vi "Get Wire Type.vi"(8 "error in (no error)":errorcluster, 11 "Message in":refnum<class "Raw Message.lvclass">) -> (0 "error out":errorcluster, 2 "Wire Type":T1, 3 "Message out":refnum<class "Raw Message.lvclass">)   [LabVIEW 2020, in "Protobuf RAW.lvlib" / "Raw Message.lvclass"]
uses:
  Raw Message.lvclass
  Type Serializer/Wire Type.ctl
  Raw Message.lvclass/Raw Message.ctl
  Wire Type Group/Wire Type Group.lvclass
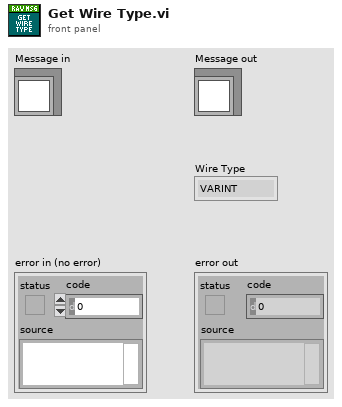
[diagram p1: front panel]
types:
  T1 = typedef "Protobuf RAW.lvlib/Wire Type Group.lvclass/Wire Type.ctl" = enum16{"VARINT", "I64", "LEN", "SGROUP", "EGROUP", "I32"}
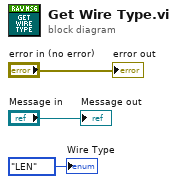
[diagram p0: block diagram]
diagram:
  "error out" <- "error in (no error)"
  "Message out" <- "Message in"
  "Wire Type" <- Wire_Type."LEN" ("Wire Type")
